vi "arduino rs232.vi"() -> ()   [LabVIEW 2014]
uses:
  <vilib>/Instr/_visa.llb/VISA Configure Serial Port (Instr).vi
panel:
  in  "stop":bool
  in  "VISA resource name":refnum<visa-resource-name>
  in  "OFF":bool
  in  "ON":bool
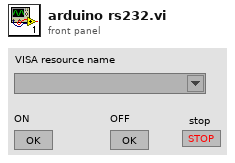
[diagram p1: front panel]
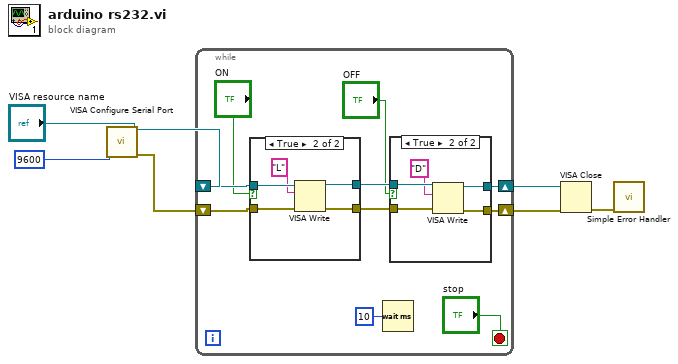
[diagram p0: block diagram]
diagram:
  n1 = call-poly "VISA Configure Serial Port"("VISA resource name"="VISA resource name", "baud rate (9600)"=u32 9600) -> ("VISA resource name out"=w5:refnum<visa-resource-name>, "error out"=w4:errorcluster)  [unwired: 12 in]
  n2 = while {
    shift-right: [w13] -> w3
    shift-left: w5 -> [w17]
    shift-right: [w12] -> w2
    shift-left: w4 -> [w16]
    stop <- "stop" stop-if-true
    n3 = case shown="True" "ON" {
      tunnel: w17 -> [w26 w31]
      tunnel: w16 -> [w25 w30]
      tunnel: [w26 w29] -> w15
      tunnel: [w25 w28] -> w14
      frame False {
      }
      frame True {
        n4 = VISA Write(VISA resource name=w31, write buffer="L", error in (no error)=w30) -> (VISA resource name out=w29:refnum<visa-resource-name>, error out=w28:errorcluster)  [unwired: 1 out]
      }
    }
    n5 = Wait (ms)(milliseconds to wait=u32 10) -> ()  [unwired: 1 out]
    n6 = case shown="True" "OFF" {
      tunnel: w15 -> [w19 w24]
      tunnel: w14 -> [w18 w23]
      tunnel: [w19 w21] -> w13
      tunnel: [w18 w20] -> w12
      frame False {
      }
      frame True {
        n7 = VISA Write(VISA resource name=w24, write buffer="D", error in (no error)=w23) -> (VISA resource name out=w21:refnum<visa-resource-name>, error out=w20:errorcluster)  [unwired: 1 out]
      }
    }
  }
  n8 = VISA Close(VISA resource name=w3, error in (no error)=w2) -> (error out=w1:errorcluster)
  n9 = call <vilib>:"Simple Error Handler.vi"("error in (no error)"=w1) -> ()  [unwired: 4 in, 5 out]
